vi "estimation_tf_motor.vi"() -> ()   [LabVIEW 2025]
uses:
  <vilib>/Analysis/7linalg.llb/Real Transpose Matrix.vi
  <vilib>/Utility/file.llb/Read Delimited Spreadsheet (DBL).vi
  <vilib>/Utility/file.llb/Write Delimited Spreadsheet (DBL).vi
  <vilib>/Analysis/NI_AALPro.lvlib
panel:
  out "Waveform Chart":dynamicdata(graph)
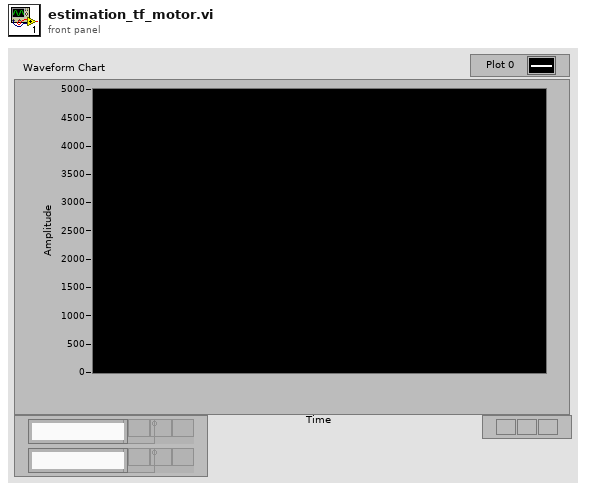
[diagram p1: front panel]
types:
  T1 = typedef "NI_Matrix.lvlib/RealMatrix.ctl" = dbl[][]
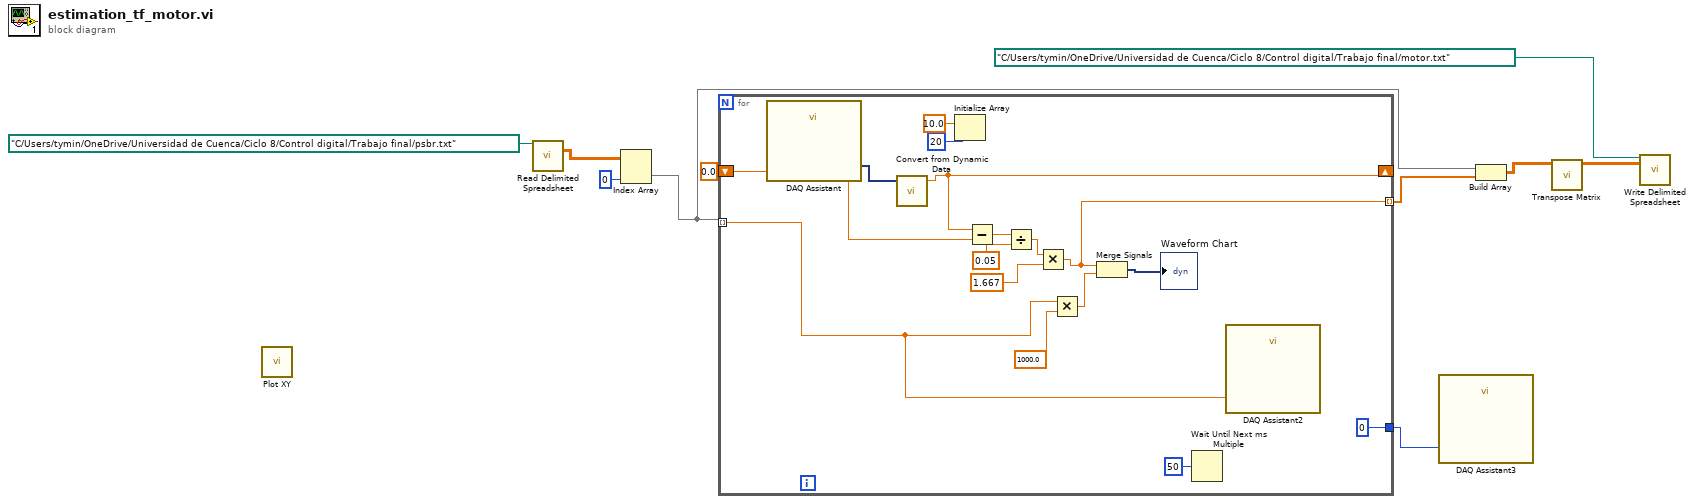
[diagram p0: block diagram]
diagram:
  n1 = call <vilib>:"Plot XY.vi"() -> ()  [unwired: 15 in, 1 out]
  n2 = call-poly <vilib>:"Read Delimited Spreadsheet.vi"("file path (dialog if empty)"=path "C:/Users/tymin/OneDrive/Universidad de Cuenca/Ciclo 8/Control digital/Trabajo final/psbr.txt") -> ("all rows"=w9:dbl[][])  [unwired: 9 in, 5 out]
  n3 = Index Array(array=w9, index (col)=0 ("disabled index (col)")) -> (element=w5:dbl[])  [unwired: 1 in]
  n4 = for {
    tunnel: w5 -> [w13] mode=indexing
    shift-right: [w24] -> _
    shift-left: 0.0 ("Scalar") -> [w25]
    tunnel: [0] -> w1
    tunnel: [w15] -> w6 mode=indexing
    n5 = call "DAQ Assistant"() -> ("data"=w14:dynamicdata)  [unwired: 16 in, 3 out]
    n6 = call "Convert from Dynamic Data"("Dynamic Data Type"=w14) -> ("Scalar"=w24:dbl)  [unwired: 3 in]
    n7 = Initialize Array(10.0 ("element"), 20 ("dimension size")) -> ()  [unwired: 1 out]
    n8 = Subtract(x=w24, y=w25) -> (x-y=w23:dbl)
    n9 = Divide(x=w23, y=0.05) -> (x/y=w21:dbl)
    n10 = Multiply(x=w21, y=1.667) -> (x*y=w15:dbl)
    n11 = Multiply(x=w13, y=1000.0) -> (x*y=w17:dbl)
    n12 = Merge Signals(w15, w17) -> (→"Waveform Chart":dynamicdata)
    n13 = Wait Until Next ms Multiple(millisecond multiple=u32 50) -> ()  [unwired: 1 out]
    n14 = call "DAQ Assistant2"("data"=w13) -> ()  [unwired: 17 in, 2 out]
  }
  n15 = call "DAQ Assistant3"("data"=w1) -> ()  [unwired: 17 in, 2 out]
  n16 = Build Array(w5, w6) -> (w4:dbl[][])
  n17 = call-poly <vilib>:"Transpose Matrix.vi"("Input Matrix"=w4) -> ("Matrix Transpose"=w3:T1)  [unwired: 9 in, 1 out]
  n18 = call-poly <vilib>:"Write Delimited Spreadsheet.vi"("file path (dialog if empty)"=path "C:/Users/tymin/OneDrive/Universidad de Cuenca/Ciclo 8/Control digital/Trabajo final/motor.txt", "2D data"=w3) -> ()  [unwired: 12 in, 2 out]
